vi "process_add_sub.vi"(10 "expression":string) -> (1 "position":u16, 2 "value":dbl)   [LabVIEW 2021]
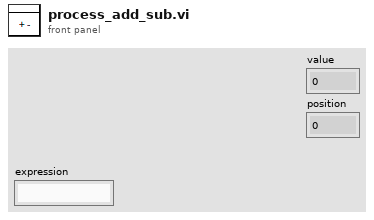
[diagram p1: front panel]
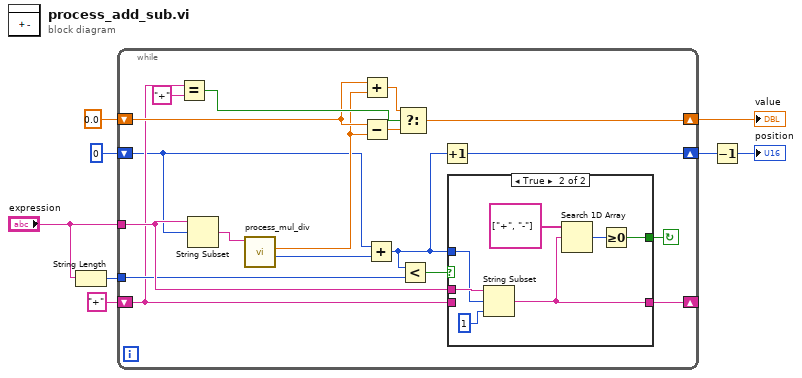
[diagram p0: block diagram]
diagram:
  n1 = String Length(string="expression") -> (length=w7:i32)
  n2 = while {
    tunnel: w7 -> [w16]
    shift-right: [w18] -> w6
    shift-left: 0.0 -> [w21]
    shift-right: [w13] -> w2
    shift-left: u16 0 ("position") -> [w9]
    tunnel: "expression" -> [w26]
    shift-right: [w11] -> _
    shift-left: "+" -> [w10]
    stop <- w12 continue-if-true
    n3 = Equal?(x=w10, y="+") -> (x = y?=w23:bool)
    n4 = String Subset(string=w26, offset (0)=w9) -> (substring=w25:string)  [unwired: 1 in]
    n5 = call "process_mul_div.vi"("expression"=w25) -> ("position"=w17:u16, "value"=w20:dbl)  [unwired: 9 in]
    n6 = Add(x=w21, y=w20) -> (x+y=w22:dbl)
    n7 = Subtract(x=w21, y=w20) -> (x-y=w19:dbl)
    n8 = Add(x=w9, y=w17) -> (x+y=w14:u16)
    n9 = Select(t=w22, s=w23, f=w19) -> (s? t:f=w18:dbl)
    n10 = Less?(x=w14, y=w16) -> (x < y?=w15:bool)
    n11 = Increment(x=w14) -> (x+1=w13:u16)
    n12 = case shown="True" w15 {
      selector: w15 -> [w28 _]
      tunnel: w26 -> [_ w32]
      tunnel: w14 -> [_ w31]
      tunnel: [w28 w33] -> w12
      tunnel: [w27 w29] -> w11
      tunnel: w10 -> [w27 _]
      frame False {
      }
      frame True {
        n13 = String Subset(string=w32, offset (0)=w31, length (rest)=1 ("offset (0)")) -> (substring=w29:string)
        n14 = Search 1D Array(1D array=string[] ["+", "-"], element=w29) -> (index of element=w34:i32)  [unwired: 1 in]
        n15 = Greater Or Equal To 0?(x=w34) -> (x >= 0?=w33:bool)
      }
    }
  }
  "value" <- w6
  n16 = Decrement(x=w2) -> (x-1=→"position":u16)
